vi "ArrayOfDropletDBs-GFV.vi"(8 "error in (no error)":errorcluster, 10 "?":T1=enum."AddDropletDB", 11 "Data in":variant) -> (0 "error out":errorcluster, 3 "Data out":variant)   [LabVIEW 2013]
doc: "Use this template to build a VI to use as a subVI."
uses:
  ArrayOfDropletDB.ctl
  DropletDB.ctl
  ArrayofDropletsDBEnum.ctl
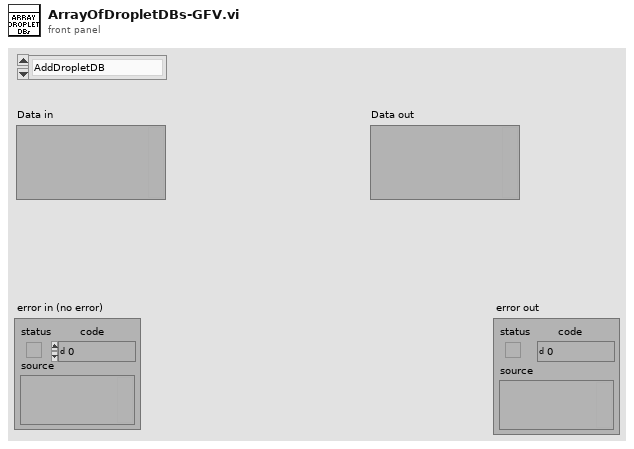
[diagram p1: front panel]
types:
  T1 = typedef "ArrayofDropletsDBEnum.ctl" = enum16{"AnalyzeDropletDBs", "AddDropletDB", "InitArrayOfDropletDB"}
  T2 = typedef "ArrayOfDropletDB.ctl" = cluster{"DropletArray":cluster{"ImageFreezeIndex":i32, "DropIndex":i32, "Position":cluster{"x":sgl, "y":sgl}, "Bounding Box":cluster{"x":sgl, "y":sgl}[], "Score":sgl, "GreyLevelInBoundingBox":dbl[], "GLDifference":dbl[], "Baseline level":dbl, "Peak":cluster{"Value":dbl, "Index":u32}, "Peak Onset":cluster{"Value":dbl, "Index":u32}, "FreezeFileName":string, "FreezeAbsTime":timestamp, "FreezeTemperature":dbl, "ImageIndexArray":u32[], "Freeze Point Found":bool, "Baseline std":dbl, "FreezedImageArray":cluster{"Image":u8[][]}[], "Include Droplet":bool, "Remark":string, "Freeze Rel Time":u32[]}[]}[]
  T3 = typedef "DropletDB.ctl" = cluster{"ImageFreezeIndex":i32, "DropIndex":i32, "Position":cluster{"x":sgl, "y":sgl}, "Bounding Box":cluster{"x":sgl, "y":sgl}[], "Score":sgl, "GreyLevelInBoundingBox":dbl[], "GLDifference":dbl[], "Baseline level":dbl, "Peak":cluster{"Value":dbl, "Index":u32}, "Peak Onset":cluster{"Value":dbl, "Index":u32}, "FreezeFileName":string, "FreezeAbsTime":timestamp, "FreezeTemperature":dbl, "ImageIndexArray":u32[], "Freeze Point Found":bool, "Baseline std":dbl, "FreezedImageArray":cluster{"Image":u8[][]}[], "Include Droplet":bool, "Remark":string, "Freeze Rel Time":u32[]}[]
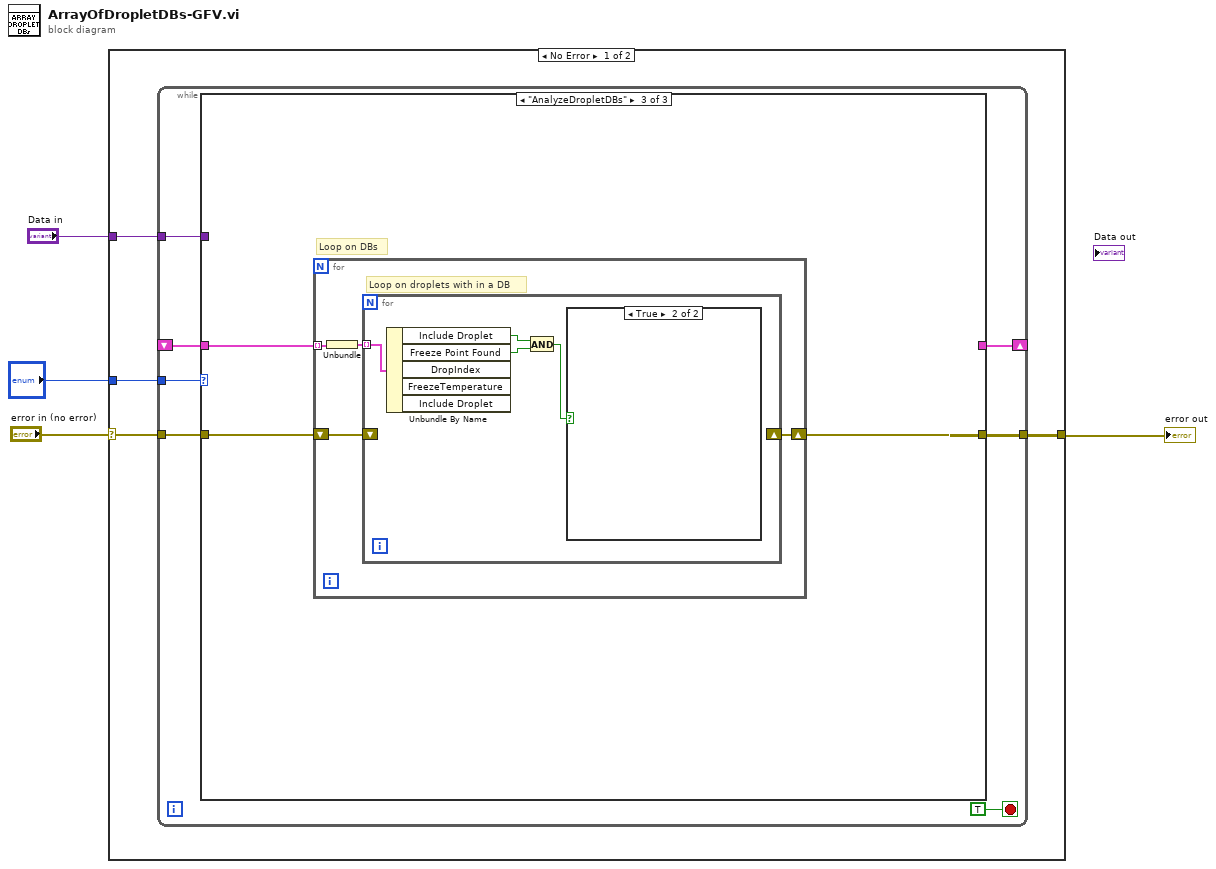
[diagram p0: block diagram]
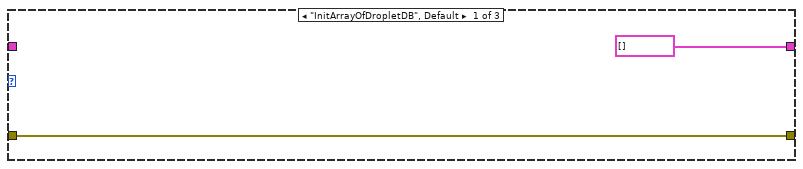
[diagram p2: hidden frame]
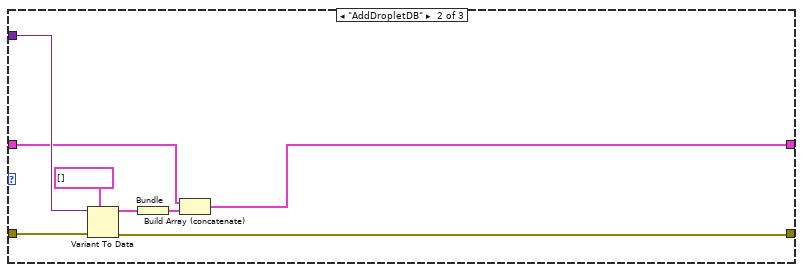
[diagram p3: hidden frame]
diagram:
  n1 = case shown="No Error" "error in (no error)" {
    selector: "error in (no error)" -> [w6 w37]
    tunnel: [w7 w37] -> w3
    tunnel: "?" -> [w8 _]
    tunnel: "Data in" -> [w5 _]
    frame No Error {
      n2 = while {
        tunnel: w8 -> [w14]
        shift-right: [w13] -> _
        shift-left: _ -> [w9]
        tunnel: [w12] -> w7
        tunnel: w6 -> [w11]
        tunnel: w5 -> [w10]
        stop <- TRUE stop-if-true
        n3 = case shown="\"AnalyzeDropletDBs\"" w14 {
          tunnel: [T2 [] ("Array of Droplets DB") w20 _] -> w13
          tunnel: [w16 w18 w26] -> w12
          tunnel: w11 -> [w16 w19 w27]
          tunnel: w10 -> [_ w25 _]
          tunnel: w9 -> [_ w21 w28]
          frame "InitArrayOfDropletDB", Default {
          }
          frame "AddDropletDB" {
            n4 = Variant To Data(error in=w19, type=T3 [] ("DropletArray"), Variant=w25) -> (data=w23:T3, error out=w18:errorcluster)
            n5 = Bundle("DropletArray"=w23) -> (w22:cluster{"DropletArray":T3})  [unwired: 1 in]
            n6 = Build Array (concatenate)(w21, w22) -> (w20:cluster{"DropletArray":T3}[])
          }
          frame "AnalyzeDropletDBs" {
            # "Loop on DBs"
            n7 = for {
              tunnel: w28 -> [w30] mode=indexing
              shift-right: [w31] -> w26
              shift-left: w27 -> [w32]
              # "Loop on droplets with in a DB"
              n8 = Unbundle(w30) -> ("DropletArray"=w29:T3)
              n9 = for {
                shift-right: [_] -> w31
                shift-left: w32 -> [_]
                tunnel: w29 -> [w36] mode=indexing
                n10 = Unbundle By Name(w36) -> ("Include Droplet"=w35:bool, "Freeze Point Found"=w34:bool)  [unwired: 3 out]
                n11 = And(x=w35, y=w34) -> (x .and. y?=w33:bool)
                n12 = case shown="True" w33 {
                  frame False {
                  }
                  frame True {
                  }
                }
              }
            }
          }
        }
      }
    }
    frame Error {
    }
  }
  "error out" <- w3
